vi "NMRsweep.vi"(0 "Center Freq (MHz)":dbl, 2 "Freq Span (MHz)":dbl, 3 "RF Level (dBm)":dbl, 4 "Foffset (MHz)":dbl, 5 "Step Width (MHz)":dbl, 6 "Sweep Mode":u16, 7 "GPIB Addr (28)":refnum<visa-resource-name>) -> (1 "error out":errorcluster)   [LabVIEW 2013]
panel:
  # "The big kahuna to setup the frequency sweep\nand amplitude"
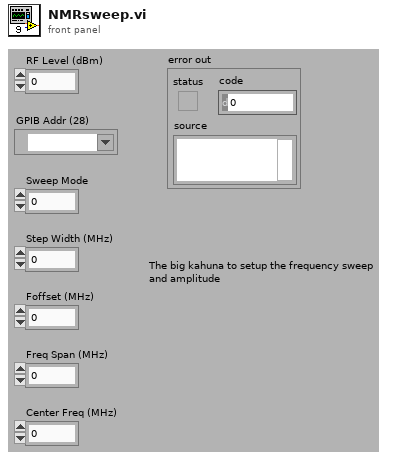
[diagram p1: front panel]
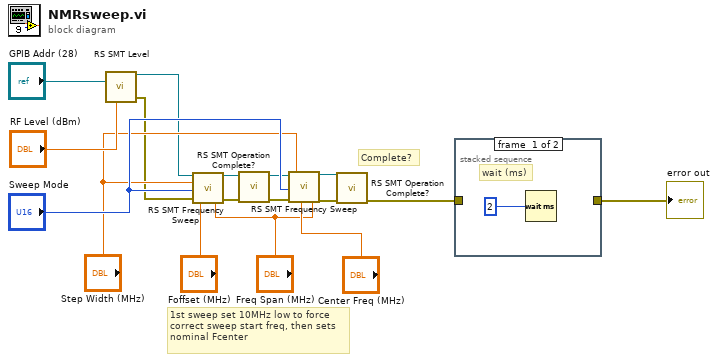
[diagram p0: block diagram]
diagram:
  # "1st sweep set 10MHz low to force \ncorrect sweep start freq, then sets\nnominal Fcenter"
  # "Complete?"
  n1 = call "RS SMT Level.vi"("VISA session"="GPIB Addr (28)", "Level (-30.0)"="RF Level (dBm)") -> ("dup VISA session"=w4:refnum<visa-resource-name>, "error out"=w3:errorcluster)  [unwired: 12 in]
  n2 = call "RS SMT Frequency Sweep.vi"("VISA session"=w4, "Sweep Mode (0:Off)"="Sweep Mode", "error in (no error)"=w3, "Step Width (MHz)"="Step Width (MHz)", "Center Freq (MHz)"="Foffset (MHz)", "Freq Span (MHz)"="Freq Span (MHz)") -> ("dup VISA session"=w6:refnum<visa-resource-name>, "error out"=w7:errorcluster)  [unwired: 12 in]
  n3 = call "RS SMT Operation Complete?.vi"("error in (no error)"=w7, "VISA session"=w6) -> ("error out"=w10:errorcluster, "dup VISA session"=w8:refnum<visa-resource-name>)  [unwired: 8 in]
  n4 = call "RS SMT Frequency Sweep.vi"("VISA session"=w8, "Sweep Mode (0:Off)"="Sweep Mode", "error in (no error)"=w10, "Step Width (MHz)"="Step Width (MHz)", "Center Freq (MHz)"="Center Freq (MHz)", "Freq Span (MHz)"="Freq Span (MHz)") -> ("dup VISA session"=w9:refnum<visa-resource-name>, "error out"=w11:errorcluster)  [unwired: 12 in]
  n5 = call "RS SMT Operation Complete?.vi"("error in (no error)"=w11, "VISA session"=w9) -> ("error out"=w2:errorcluster)  [unwired: 8 in, 1 out]
  n6 = stacked-sequence {
    tunnel: w2 -> [_ w19]
    tunnel: [_ w19] -> w1
    frame #0 {
      # "wait (ms)"
      n7 = Wait (ms)(milliseconds to wait=2) -> ()  [unwired: 1 out]
    }
    frame #1 {
    }
  }
  "error out" <- w1
